vi "Lightning Periodic Tasks.vi"   [LabVIEW 2015]
uses:
  <vilib>/Platform/TimedLoop/XDataNode/timing_clust.ctl
  <vilib>/Platform/TimedLoop/XDataNode/nitl_modes.ctl
  <vilib>/Platform/TimedLoop/XDataNode/wakeup.ctl
  <vilib>/Rock Robotics/WPI/DriverStation/WPI_DriverStationRobotMode2.ctl
  Robot Global Data.vi
  <vilib>/platform/TimedLoop/XDataNode/XDataNode.xnode
  <vilib>/Platform/TimedLoop/XDataNode/XDNodeRunTimeDep.lvlib
types:
  T1 = typedef "XDNodeRunTimeDep.lvlib/timing_clust.ctl" = cluster{"Expected End [f-1]":u64, "Actual End [f-1]":u64, "Finished Late? [f-1]":bool, "Expected End [i-1]":u64, "Actual End [i-1]":u64, "Finished Late? [i-1]":bool, "Expected Start [i]":u64, "Actual Start [i]":u64, "Expected Start [f]":u64, "Actual Start [f]":u64, "Source Name":string, "Structure Name":string, "Period":i64, "Deadline":i64, "Offset":i64, "Start":i64, "Priority":i32, "Timeout":i32, "Mode":T2, "Wakeup Reason":T3, "Error":errorcluster, "Source Type":string, "Secondary Source Type":string, "Global End Time":u64, "Global Start Time":u64, "Frame Duration":u64, "Iteration Duration":u64, "Assigned CPU":i32, "I/O Scan Engine Mode":u32}
  T2 = typedef "XDNodeRunTimeDep.lvlib/nitl_modes.ctl" = enum32{"No Change", "Process missed periods, maintain original phase", "Discard missed periods, maintain original phase", "Process missed periods, ignore original phase", "Discard missed periods, ignore original phase"}
  T3 = typedef "XDNodeRunTimeDep.lvlib/wakeup.ctl" = enum32{"Normal", "Aborted", "Asynchronous wakeup", "Timing source error", "Timed loop error", "Timeout"}
  T4 = typedef "WPI_DriverStationRobotMode2.ctl" = enum16{"Autonomous Disabled", "Autonomous Enabled", "Teleop Disabled", "Teleop Enabled", "Disconnected", "Finish", "Test Disabled", "Test Enabled", "Emergency Stopped"}
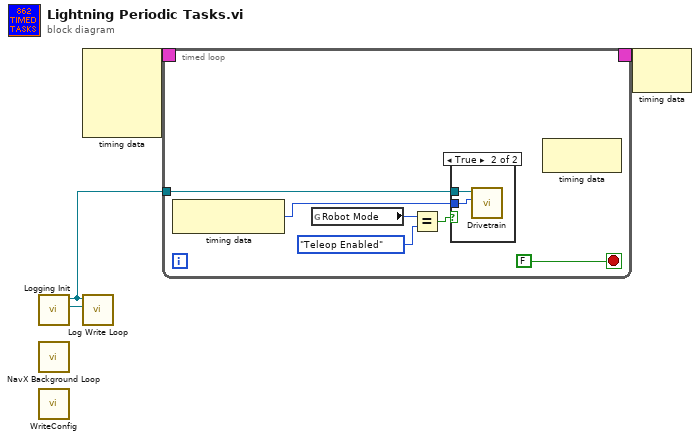
[diagram p0: block diagram]
diagram:
  n1 = call "Logging Init.vi"() -> ("Logging Reference"=w1:refnum<file>, "Logging FIFO"=w2:refnum<k33>)  [unwired: 9 in, 1 out]
  n2 = call "NavX Background Loop.vi"() -> ()  [unwired: 12 in]
  n3 = call "WriteConfig.vi"() -> ()  [unwired: 12 in]
  n4 = node-c288() -> (w4:T1)  [unwired: 4 in]
  n5 = call "Log Write Loop.vi"("Logging FIFO"=w2, "Byte Stream File in"=w1) -> ()  [unwired: 8 in]
  n6 = timed-loop {
    tunnel: w2 -> [w10]
    timing: w4 -> [_]
    timing-out: [_] -> w3
    stop <- FALSE stop-if-true
    n7 = node-c288() -> (w8:i64)  [unwired: 1 in]
    n8 = global read "Robot Global Data.vi" "Robot Mode"() -> (w6:T4)
    n9 = Equal?(x=w6, y=WPI_DriverStationRobotMode2."Teleop Enabled") -> (x = y?=w5:bool)
    n10 = case shown="True" w5 {
      tunnel: w10 -> [_ w12]
      tunnel: w8 -> [_ w11]
      frame False {
      }
      frame True {
        n11 = call "Drivetrain.vi"("Duration"=w11, "rt fifo"=w12) -> ()  [unwired: 10 in]
      }
    }
    n12 = node-c288() -> ()  [unwired: 1 in, 1 out]
  }
  n13 = node-c288(w3) -> ()  [unwired: 1 out]
